vi "is_initialized.vi"(8 "error in (no error)":errorcluster, 11 "FPGAWrapperMH120124FrameScan_PXI7813R in":refnum<class "FPGAWrapperMH120124FrameScan_PXI7813R.lvclass">) -> (0 "error out":errorcluster, 2 "is initialized?":bool, 3 "FPGAWrapperMH120124FrameScan_PXI7813R out":refnum<class "FPGAWrapperMH120124FrameScan_PXI7813R.lvclass">)   [LabVIEW 2010, in "FPGAWrapperMH120124FrameScan_PXI7813R.lvclass"]
uses:
  FPGAWrapperMH120124FrameScan_PXI7813R.lvclass
  class_data.vi
  common/classes/ErrorController/ErrorController/class_data.vi
  common/classes/ErrorController/ErrorController/ErrorController.lvclass
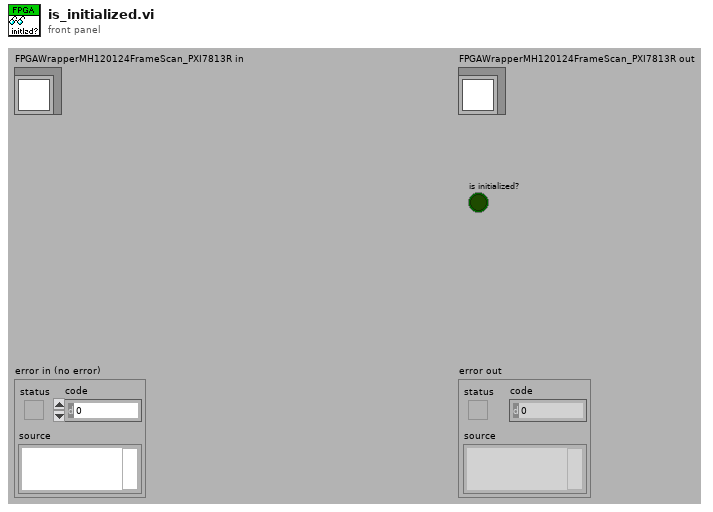
[diagram p1: front panel]
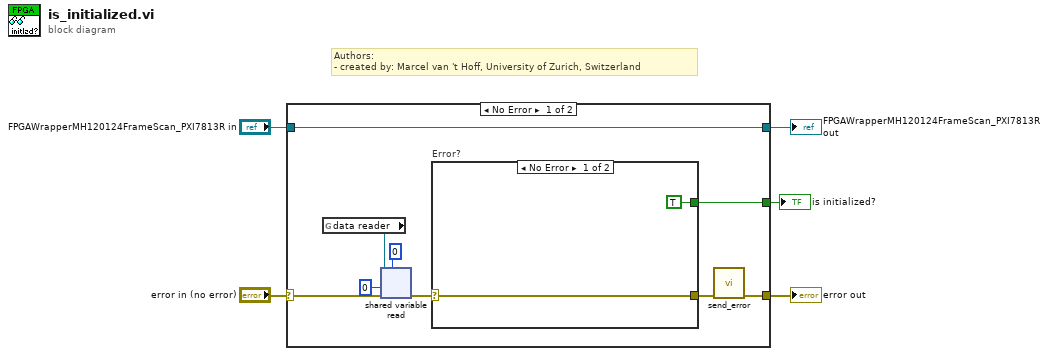
[diagram p0: block diagram]
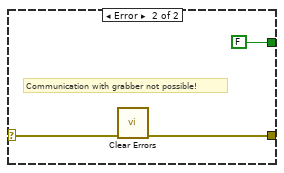
[diagram p2: hidden frame]
diagram:
  # "Authors: \n- created by: Marcel van 't Hoff, University of Zurich, Switzerland"
  n1 = case shown="No Error" "error in (no error)" {
    selector: "error in (no error)" -> [w10 w21]
    tunnel: [w7 w21] -> w4
    tunnel: [w14 w20] -> w2
    tunnel: "FPGAWrapperMH120124FrameScan_PXI7813R in" -> [w14 w20]
    tunnel: [w8 _] -> w1
    frame No Error {
      n2 = global read "class_data.vi" "data reader"() -> (w11:refnum<k21>)
      n3 = shared-variable-read(w11, w10, 0 ("timeout in ms (-1)"), 0 ("# elements (-1)")) -> (w9:errorcluster)  [unwired: 3 out]
      n4 = case "Error?" shown="No Error" w9 {
        selector: w9 -> [w16 w18]
        tunnel: [TRUE FALSE] -> w8
        tunnel: [w16 w17] -> w6
        frame No Error {
        }
        frame Error {
          # "Communication with grabber not possible!"
          n5 = call <vilib>:"Clear Errors.vi"("error in (no error)"=w18) -> ("error out"=w17:errorcluster)  [unwired: 6 in]
        }
      }
      n6 = call "send_error.vi"("error in (no error)"=w6) -> ("error out"=w7:errorcluster)  [unwired: 10 in]
    }
    frame Error {
    }
  }
  "error out" <- w4
  "FPGAWrapperMH120124FrameScan_PXI7813R out" <- w2
  "is initialized?" <- w1
